vi "Get Test Suite.vi"(7 "MsgSerializer":refnum<class "MsgSerializer.lvclass">, 9 "ID":i32, 10 "Node Result":T5) -> (2 "Test Suite":T1)   [LabVIEW 2013, in "JUnit for Azure Pipelines.lvclass"]
uses:
  JUnit for Azure Pipelines.lvclass
  <vilib>/addons/_JKI Toolkits/Caraya/classes/Test Result/Node Results (Extended).ctl
  <vilib>/addons/_JKI Toolkits/Caraya/classes/Test Result/Test Node (Extended).ctl
  <vilib>/addons/_JKI Toolkits/Caraya/classes/Test Result/Test Registration Data.ctl
  <vilib>/addons/_JKI Toolkits/Caraya/classes/Test Result/Assert Event Data (Extended).ctl
  Test Suite.ctl
  Test Case.ctl
  Test Result.ctl
  Test Case Property.ctl
  <vilib>/addons/_JKI Toolkits/Caraya/classes/MsgSerializer/MsgSerializer.lvclass
  <vilib>/addons/_JKI Toolkits/Caraya/classes/Test Result/Test Result.lvclass
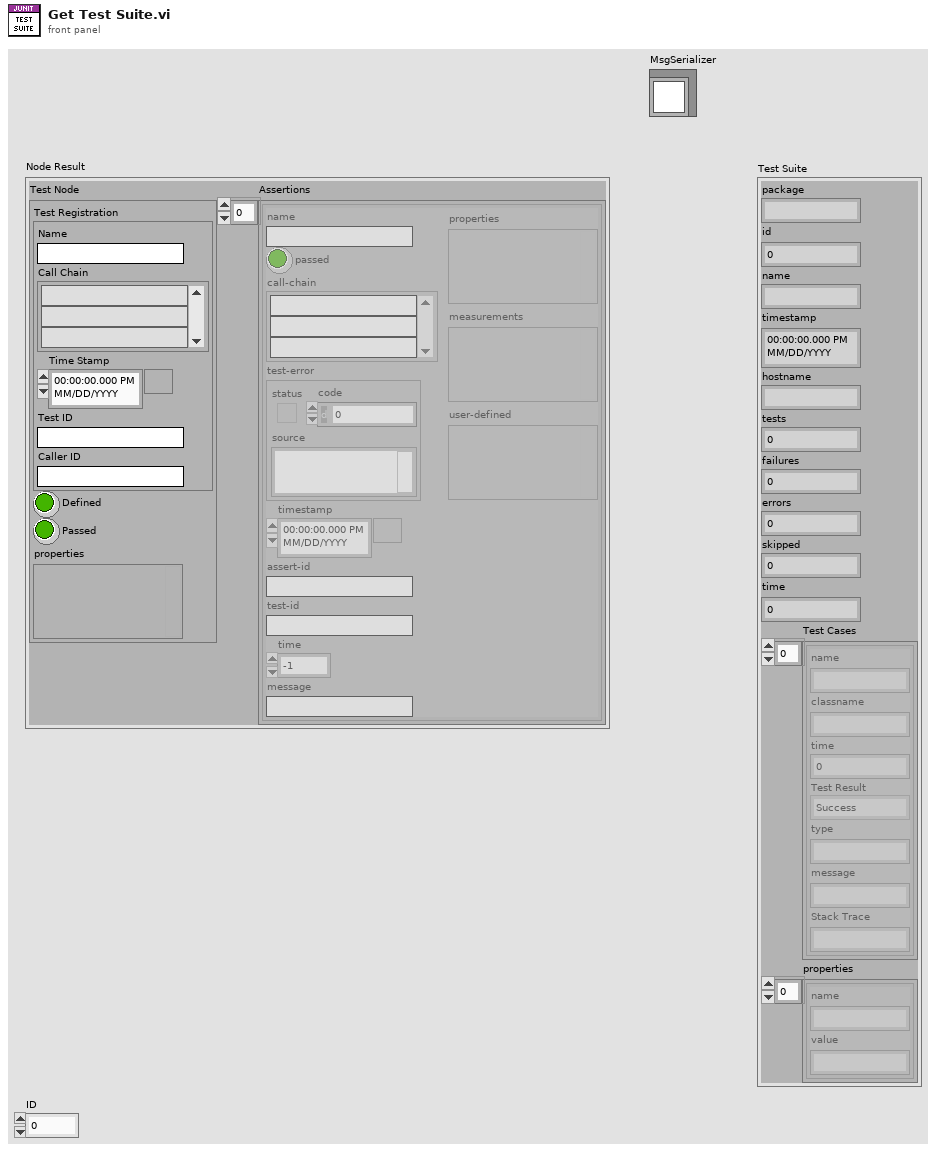
[diagram p1: front panel]
types:
  T1 = typedef "JUnit for Azure Pipelines.lvclass/Test Suite.ctl" = cluster{"package":string, "id":i32, "name":string, "timestamp":timestamp, "hostname":string, "tests":i32, "failures":i32, "errors":i32, "skipped":i32, "time":dbl, "Test Cases":T2[], "properties":T4[]}
  T2 = typedef "JUnit for Azure Pipelines.lvclass/Test Case.ctl" = cluster{"name":string, "classname":string, "time":dbl, "Test Result":T3, "type":string, "message":string, "Stack Trace":string}
  T3 = typedef "JUnit for Azure Pipelines.lvclass/Test Result.ctl" = enum16{"Success", "Failure", "Error", "Skipped"}
  T4 = typedef "JUnit for Azure Pipelines.lvclass/Test Case Property.ctl" = cluster{"name":string, "value":string}
  T5 = typedef "Caraya.lvlib/Test Result.lvclass/Node Results (Extended).ctl" = cluster{"Test Node":T6, "Assertions":T8[]}
  T6 = typedef "Caraya.lvlib/Test Result.lvclass/Test Node (Extended).ctl" = cluster{"Test Registration":T7, "Defined":bool, "Passed":bool, "properties":variant}
  T7 = typedef "Caraya.lvlib/Test Result.lvclass/Test Registration Data.ctl" = cluster{"Name":string, "Call Chain":string[], "Time Stamp":timestamp, "Test ID":string, "Caller ID":string}
  T8 = typedef "Caraya.lvlib/Test Result.lvclass/Assert Event Data (Extended).ctl" = cluster{"name":string, "passed":bool, "call-chain":string[], "test-error":errorcluster, "timestamp":timestamp, "assert-id":string, "test-id":string, "time":dbl, "message":string, "properties":variant, "measurements":variant, "user-defined":variant}
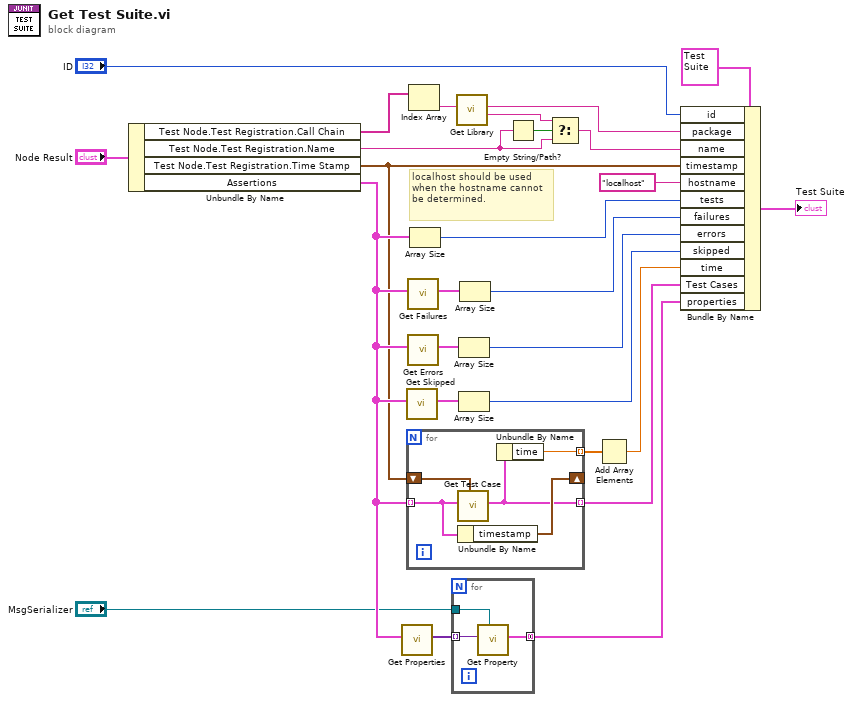
[diagram p0: block diagram]
diagram:
  # "localhost should be used when the hostname cannot be determined."
  n1 = Unbundle By Name("Node Result") -> ("Test Node.Test Registration.Call Chain"=w7:string[], "Test Node.Test Registration.Name"=w1:string, "Test Node.Test Registration.Time Stamp"=w10:timestamp, "Assertions"=w14:T8[])
  n2 = call "Get Properties.vi"("Assertions"=w14) -> ("Properties"=w13:variant[])  [unwired: 10 in]
  n3 = call "Get Skipped.vi"("Assertions"=w14) -> ("Skipped"=w24:T8[])  [unwired: 10 in]
  n4 = for {
    tunnel: w14 -> [w30] mode=indexing
    tunnel: [w29] -> w16 mode=indexing
    shift-right: [w32] -> _
    shift-left: w10 -> [w31]
    tunnel: [w28] -> w9 mode=indexing
    n5 = call "Get Test Case.vi"("Start Time"=w31, "Assert Event Data"=w30) -> ("Test Case"=w29:T2)  [unwired: 9 in]
    n6 = Unbundle By Name(w30) -> ("timestamp"=w32:timestamp)
    n7 = Unbundle By Name(w29) -> ("time"=w28:dbl)
  }
  n8 = call "Get Failures.vi"("Assertions"=w14) -> ("Failures"=w26:T8[])  [unwired: 10 in]
  n9 = call "Get Errors.vi"("Assertions"=w14) -> ("Errors"=w25:T8[])  [unwired: 10 in]
  n10 = Index Array(array=w7) -> (element=w6:string)  [unwired: 1 in]
  n11 = Array Size(array=w14) -> (size(s)=w22:i32)
  n12 = for {
    tunnel: w13 -> [w35] mode=indexing
    tunnel: "MsgSerializer" -> [w34]
    tunnel: [w33] -> w11 mode=concatenating
    n13 = call "Get Property.vi"("MsgSerializer"=w34, "Property"=w35) -> ("Properties"=w33:T4[])  [unwired: 9 in]
  }
  n14 = call "Get Library.vi"("Call Chain"=w6) -> ("Name"=w3:string, "Package"=w5:string)  [unwired: 9 in]
  n15 = Array Size(array=w25) -> (size(s)=w20:i32)
  n16 = Array Size(array=w24) -> (size(s)=w19:i32)
  n17 = Array Size(array=w26) -> (size(s)=w21:i32)
  n18 = Empty String/Path?(string/path=w1) -> (empty?=w4:bool)
  n19 = Select(t=w3, s=w4, f=w1) -> (s? t:f=w2:string)
  n20 = Add Array Elements(numeric array=w9) -> (sum=w8:dbl)
  n21 = Bundle By Name(cluster=T1 {"package"="", "id"=0, "name"="", "timestamp"=timestamp(0 s since 1904-01-01), "hostname"="", "tests"=0, "failures"=0, "errors"=0, "skipped"=0, "time"=0.0, "Test Cases"=[], "properties"=[]} ("Test Suite"), "id"="ID", "package"=w5, "name"=w2, "timestamp"=w10, "hostname"="localhost", "tests"=w22, "failures"=w21, "errors"=w20, "skipped"=w19, "time"=w8, "Test Cases"=w16, "properties"=w11) -> (→"Test Suite":T1)
